vi "Requests.vi"(8 "error in (no error)":errorcluster, 9 "write enable":bool=TRUE, 11 "ICPCON ET7024 in":refnum<class "ICPCON ET-7024.lvclass">) -> (0 "error out":errorcluster, 3 "ICPCON ET7024 out":refnum<class "ICPCON ET-7024.lvclass">)   [LabVIEW 2021, in "ICPCON ET-7024.lvclass"]
uses:
  ICPCON ET-7024.lvclass
  D:/my_projects/projects/Algorithms/Labview/21/Modbus_v121c/Network Protocol/MB/Modbus Master CR.lvclass
  D:/my_projects/projects/Algorithms/Labview/21/Modbus_v121c/Network Protocol/Network Master/Network Master.lvclass
  MB/Modbus Master CR.lvclass/Modbus Master CR.ctl
  Modbus Data Unit/Modbus Data Unit.lvclass/Modbus Data Unit.ctl
  Network Master/Network Master.lvclass/Network Master.ctl
  Master Function Definition/Read Discrete Inputs Request.vi
  Network Master/Read write Master.vi
  Master Function Definition/Read Discrete Inputs Response.vi
  Master Function Definition/Read Holding Registers Request.vi
  Master Function Definition/Read Holding Registers Response.vi
  Master Function Definition/Write Multiple Registers Request.vi
  Master Function Definition/Function data mismatch error.vi
  Master Function Definition/Write Multiple Registers Response.vi
  Master Function Definition/Read Coils Request.vi
  Master Function Definition/Read Coils Response.vi
  Master Function Definition/Write Multiple Coils Request.vi
  Master Function Definition/Write Multiple Coils Response.vi
  Modbus Data Unit/Construct PDU.vi
  Utility/Bytes to Bits.vi
  Master Function Definition/Function code mismatch error.vi
  Data Model/Error Generator.vi
  Modbus Data Unit/Deconstruct PDU.vi
  Utility/Bytes to U16s.vi
  Utility/U16s to Bytes.vi
  Utility/Bits to Bytes.vi
  Modbus Data Unit/Modbus Data Unit.lvclass
  Data Model/Device Data Model.lvclass
  Transmission Data Unit/Transmission Data Unit.lvclass
  MB/Modbus Master CR.lvclass
  Network Master/Network Master.lvclass
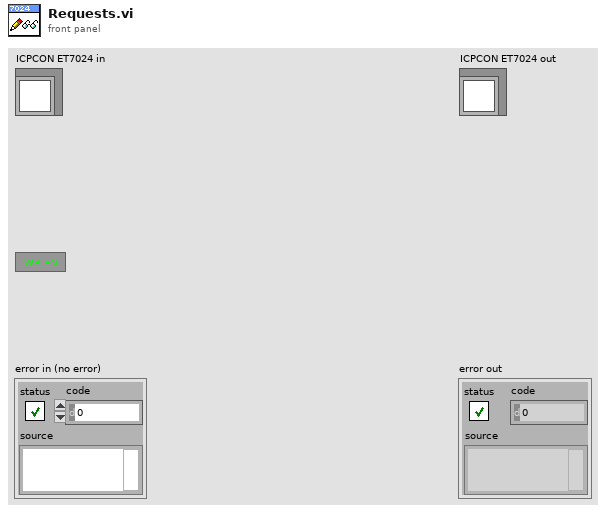
[diagram p1: front panel]
types:
  T1 = typedef "Modbus Master CR.lvclass/N channel.ctl" = cluster{"N DI channel":u16, "N DO channel":u16, "N AI channel":u16, "N AO channel":u16}
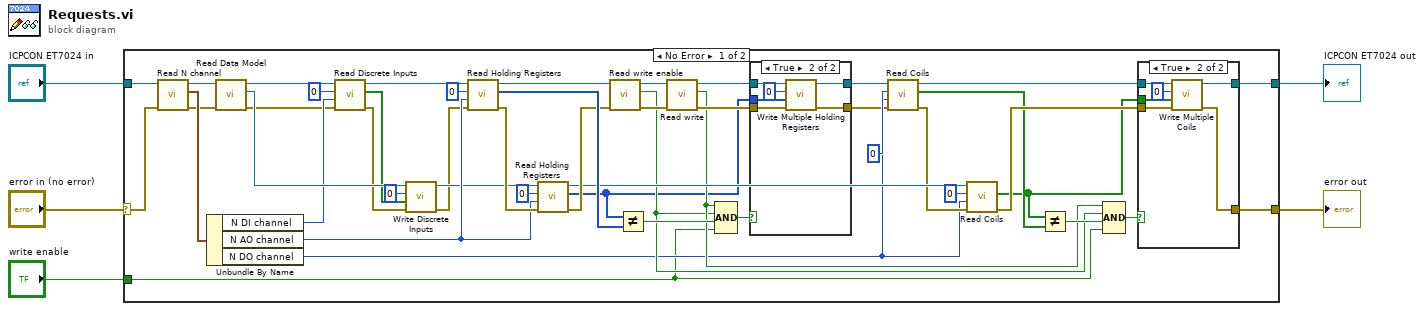
[diagram p0: block diagram]
diagram:
  n1 = case shown="No Error" "error in (no error)" {
    selector: "error in (no error)" -> [w49 w71]
    tunnel: [w13 w71] -> w3
    tunnel: [w8 w70] -> w4
    tunnel: "ICPCON ET7024 in" -> [w51 w70]
    tunnel: "write enable" -> [w14 _]
    frame No Error {
      n2 = call "Read N channel.vi"("error in (no error)"=w49, "MB_v2 in"=w51) -> ("error out"=w48:errorcluster, "N channel"=w52:T1, "MB_v2 out"=w50:refnum<class "ICPCON ET-7024.lvclass">)  [unwired: 7 in]
      n3 = Unbundle By Name(w52) -> ("N DI channel"=w33:u16, "N AO channel"=w38:u16, "N DO channel"=w16:u16)
      n4 = call "Read Data Model.vi"("error in (no error)"=w48, "MB_TCP in"=w50) -> ("error out"=w11:errorcluster, "Data Model"=w37:refnum<class "Device Data Model.lvclass">, "MB_TCP out"=w12:refnum<class "ICPCON ET-7024.lvclass">)  [unwired: 7 in]
      n5 = call "Read Discrete Inputs.vi"("error in (no error)"=w11, "number of discrete inputs"=w33, "starting address"=u16 0, "Modbus master in"=w12) -> ("error out"=w31:errorcluster, "discrete input values"=w32:bool[], "Modbus master out"=w30:refnum<class "ICPCON ET-7024.lvclass">)  [unwired: 5 in]
      n6 = call-dynamic "Write Discrete Inputs.vi"("error in (no error)"=w31, "input values"=w32, "starting address"=u16 0, "Device Data Model in"=w37) -> ("error out"=w29:errorcluster, "Device Data Model out"=w36:refnum<class "Device Data Model.lvclass">)  [unwired: 6 in]
      n7 = call "Read Holding Registers.vi"("error in (no error)"=w29, "number of holding registers"=w38, "starting address"=u16 0, "Modbus master in"=w30) -> ("error out"=w39:errorcluster, "register values"=w41:u16[], "Modbus master out"=w10:refnum<class "ICPCON ET-7024.lvclass">)  [unwired: 5 in]
      n8 = call-dynamic "Read Holding Registers.vi"("error in"=w39, "number of registers"=w38, "starting address"=u16 0, "device data model in"=w36) -> ("error out"=w40:errorcluster, "data"=w7:u16[], "device data model out"=w26:refnum<class "Device Data Model.lvclass">)  [unwired: 5 in]
      n9 = call "Read write enable.vi"("error in (no error)"=w40, "MB in"=w10) -> ("error out"=w45:errorcluster, "write enable"=w23:bool, "MB out"=w46:refnum<class "ICPCON ET-7024.lvclass">)  [unwired: 7 in]
      n10 = Not Equal?(x=w7, y=w41) -> (x != y?=w47:bool)
      n11 = call "Read write.vi"("error in (no error)"=w45, "MB in"=w46) -> ("error out"=w44:errorcluster, "Write"=w24:bool, "MB out"=w9:refnum<class "ICPCON ET-7024.lvclass">)  [unwired: 7 in]
      n12 = Compound Arithmetic op=AND(w24, w23, w47, w14) -> (w53:bool)
      n13 = case shown="True" w53 {
        tunnel: w44 -> [w55 w59]
        tunnel: [w55 w57] -> w17
        tunnel: w7 -> [_ w58]
        tunnel: w9 -> [w54 w60]
        tunnel: [w54 w56] -> w18
        frame False {
        }
        frame True {
          n14 = call "Write Multiple Holding Registers.vi"("error in (no error)"=w59, "holding register values"=w58, "starting address"=u16 0, "Modbus master in"=w60) -> ("error out"=w57:errorcluster, "Modbus master out"=w56:refnum<class "ICPCON ET-7024.lvclass">)  [unwired: 6 in]
        }
      }
      n15 = call "Read Coils.vi"("error in (no error)"=w17, "number of coils"=w16, "starting address"=u16 0, "Modbus master in"=w18) -> ("error out"=w20:errorcluster, "coil values"=w21:bool[], "Modbus master out"=w22:refnum<class "ICPCON ET-7024.lvclass">)  [unwired: 5 in]
      n16 = call-dynamic "Read Coils.vi"("error in"=w20, "number of coils"=w16, "starting address"=u16 0, "device data model in"=w26) -> ("error out"=w25:errorcluster, "data"=w6:bool[])  [unwired: 5 in, 1 out]
      n17 = Not Equal?(x=w6, y=w21) -> (x != y?=w28:bool)
      n18 = Compound Arithmetic op=AND(w24, w23, w28, w14) -> (w27:bool)
      n19 = case shown="True" w27 {
        tunnel: w25 -> [w63 w68]
        tunnel: [w63 w65] -> w13
        tunnel: w6 -> [_ w67]
        tunnel: w22 -> [w62 w69]
        tunnel: [w62 w64] -> w8
        frame False {
        }
        frame True {
          n20 = call "Write Multiple Coils.vi"("error in (no error)"=w68, "coil values"=w67, "starting address"=u16 0, "Modbus master in"=w69) -> ("error out"=w65:errorcluster, "Modbus master out"=w64:refnum<class "ICPCON ET-7024.lvclass">)  [unwired: 6 in]
        }
      }
    }
    frame Error {
    }
  }
  "error out" <- w3
  "ICPCON ET7024 out" <- w4
